vi "Get Sample Local WP.vi"   [LabVIEW 2009]
uses:
  cRIO/Functional Global Variables/Actions for FG's.ctl
  Support Files/ElementRec.ctl
  Support Files/LocalWaypointRec.ctl
types:
  T1 = typedef "ElementRec.ctl" = cluster{"ElementUID":u16, " PreviousUID":u16, " NextUID":u16, "LocalWaypointRec":T2}
  T2 = typedef "LocalWaypointRec.ctl" = cluster{"Presence Vector":u8, " X":dbl, " Y":dbl, " Z":dbl, "Roll":dbl, "Pitch":dbl, "Yaw":dbl, "Waypoint Tolerance":dbl, "Path Tolerance":dbl, "Is Active?":bool}
  T3 = typedef "Actions for FG's.ctl" = enum16{"Read", "Write"}
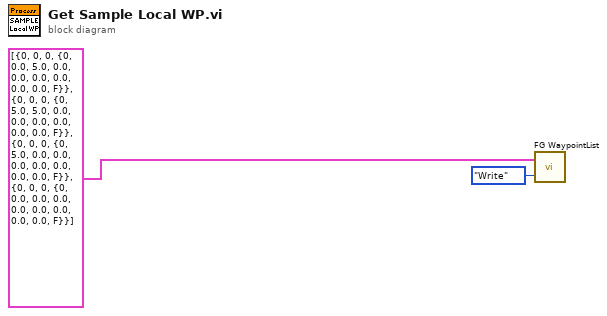
[diagram p0: block diagram]
diagram:
  n1 = call "FG WaypointList.vi"("FG Action (Read)"=Actions_for_FG's."Write", "Local Waypoint List in"=T1[] [{"ElementUID"=0, " PreviousUID"=0, " NextUID"=0, "LocalWaypointRec"={"Presence Vector"=0, " X"=0.0, " Y"=5.0, " Z"=0.0, "Roll"=0.0, "Pitch"=0.0, "Yaw"=0.0, "Waypoint Tolerance"=0.0, "Path Tolerance"=0.0, "Is Active?"=FALSE}}, {"ElementUID"=0, " PreviousUID"=0, " NextUID"=0, "LocalWaypointRec"={"Presence Vector"=0, " X"=5.0, " Y"=5.0, " Z"=0.0, "Roll"=0.0, "Pitch"=0.0, "Yaw"=0.0, "Waypoint Tolerance"=0.0, "Path Tolerance"=0.0, "Is Active?"=FALSE}}, {"ElementUID"=0, " PreviousUID"=0, " NextUID"=0, "LocalWaypointRec"={"Presence Vector"=0, " X"=5.0, " Y"=0.0, " Z"=0.0, "Roll"=0.0, "Pitch"=0.0, "Yaw"=0.0, "Waypoint Tolerance"=0.0, "Path Tolerance"=0.0, "Is Active?"=FALSE}}, {"ElementUID"=0, " PreviousUID"=0, " NextUID"=0, "LocalWaypointRec"={"Presence Vector"=0, " X"=0.0, " Y"=0.0, " Z"=0.0, "Roll"=0.0, "Pitch"=0.0, "Yaw"=0.0, "Waypoint Tolerance"=0.0, "Path Tolerance"=0.0, "Is Active?"=FALSE}}] ("Local Waypoint List in 2")) -> ()  [unwired: 1 out]
